vi "111 (SubVI).vi"(0 "scan angle":sgl=90.0, 5 "step angle":sgl=4.0, 7 "stop":bool) -> (2 "sensor":bool, 3 "x":dbl, 4 "Data Value Reference out":refnum<data-value>, 6 "left motor":bool, 8 "y":dbl, 10 "right motor":bool, 12 "Array":u32[][](array[colorbox]), 13 "velocity":dbl, 14 "sensor data":cluster{dbl[], dbl[]}(graph)={[-0.048166929668633715], [0.4724490056471417]})   [LabVIEW 2011]
uses:
  <vilib>/robotics/Navigation/shared/WorldMap/OccupancyGridWorldMap/NI_Robotics_OccupancyGridWorldMap.lvclass
  <vilib>/Platform/TimedLoop/XDataNode/timing_clust.ctl
  <vilib>/Platform/TimedLoop/XDataNode/nitl_modes.ctl
  <vilib>/Platform/TimedLoop/XDataNode/wakeup.ctl
  <vilib>/robotics/Starter Kit/2.0/9632 Host Interface/NI_Robotics_Starter Kit Host_9632_2.0.lvclass
  <vilib>/Utility/AngleManip/Degrees to Radians (Scalar SGL).vi
  <vilib>/robotics/Steering/Steering Frame/Apply Steering Frame Velocity to Motors.vi
  <vilib>/Utility/AngleManip/Degrees to Radians (Scalar DBL).vi
  <vilib>/robotics/Steering/Steering Frame/Get Steering Frame Velocity from Motors.vi
  <vilib>/Platform/TimedLoop/XDataNode/XDataNode.xnode
  <vilib>/Utility/AngleManip/NI_AngleManipulation.lvlib
  <vilib>/robotics/Utilities/Scan Angles/NI_Robotics_Scan Angles.lvlib
  <vilib>/robotics/Starter Kit/2.0/NI_Robotics_Starter Kit Host_2.0.lvlib
  <vilib>/Platform/TimedLoop/XDataNode/XDNodeRunTimeDep.lvlib
  <vilib>/robotics/Starter Kit/Host Interface/NI_Robotics_Starter Kit Host.lvclass
  <vilib>/robotics/Steering/Steering Frame/NI_Robotics_Steering Frame.lvclass
  <vilib>/ptbypt/NI_PtbyPt.lvlib
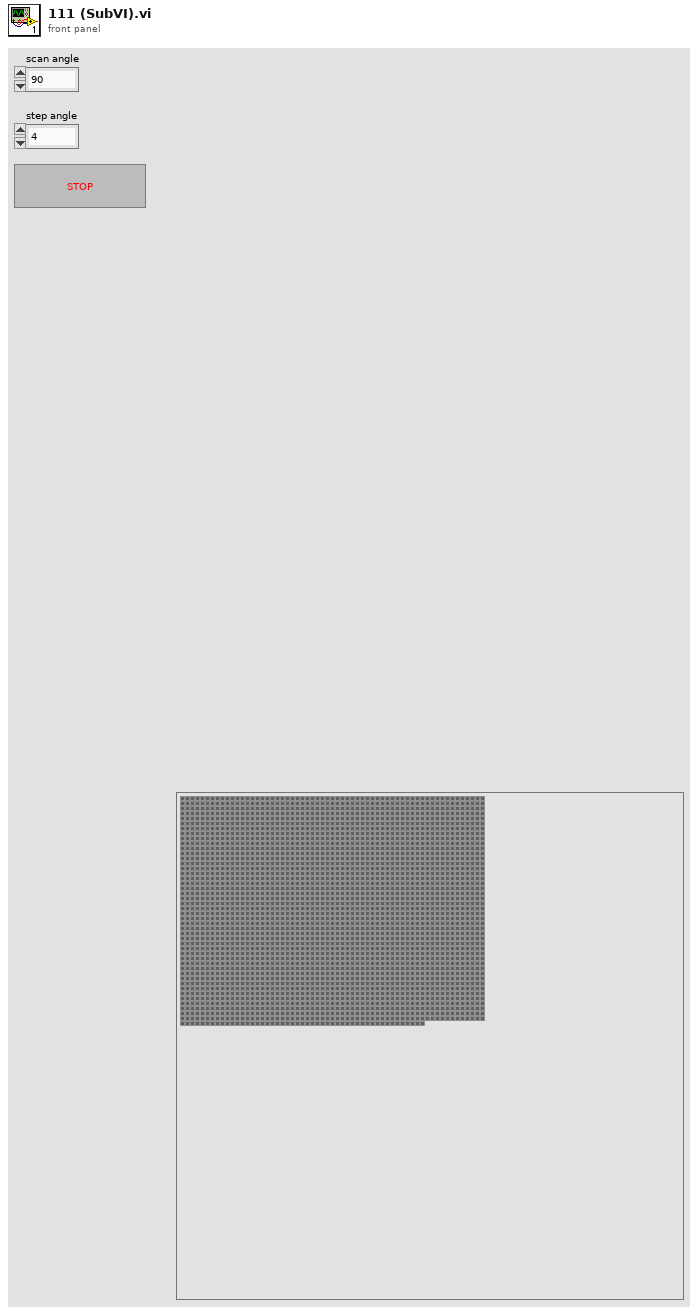
[diagram p1: front panel]
types:
  T1 = typedef "NI_Robotics_Scan Angles.lvlib/Scan Angle Data.ctl" = cluster{"angles":dbl[], "distances":dbl[], "current index":i32, "previous index":i32}
  T2 = typedef "XDNodeRunTimeDep.lvlib/timing_clust.ctl" = cluster{"Expected End [f-1]":u64, "Actual End [f-1]":u64, "Finished Late? [f-1]":bool, "Expected End [i-1]":u64, "Actual End [i-1]":u64, "Finished Late? [i-1]":bool, "Expected Start [i]":u64, "Actual Start [i]":u64, "Expected Start [f]":u64, "Actual Start [f]":u64, "Source Name":string, "Structure Name":string, "Period":i64, "Deadline":i64, "Offset":i64, "Start":i64, "Priority":i32, "Timeout":i32, "Mode":T3, "Wakeup Reason":T4, "Error":errorcluster, "Source Type":string, "Secondary Source Type":string, "Global End Time":u64, "Global Start Time":u64, "Frame Duration":u64, "Iteration Duration":u64, "Assigned CPU":i32, "I/O Scan Engine Mode":u32}
  T3 = typedef "XDNodeRunTimeDep.lvlib/nitl_modes.ctl" = enum32{"No Change", "Process missed periods, maintain original phase", "Discard missed periods, maintain original phase", "Process missed periods, ignore original phase", "Discard missed periods, ignore original phase"}
  T4 = typedef "XDNodeRunTimeDep.lvlib/wakeup.ctl" = enum32{"Normal", "Aborted", "Asynchronous wakeup", "Timing source error", "Timed loop error", "Timeout"}
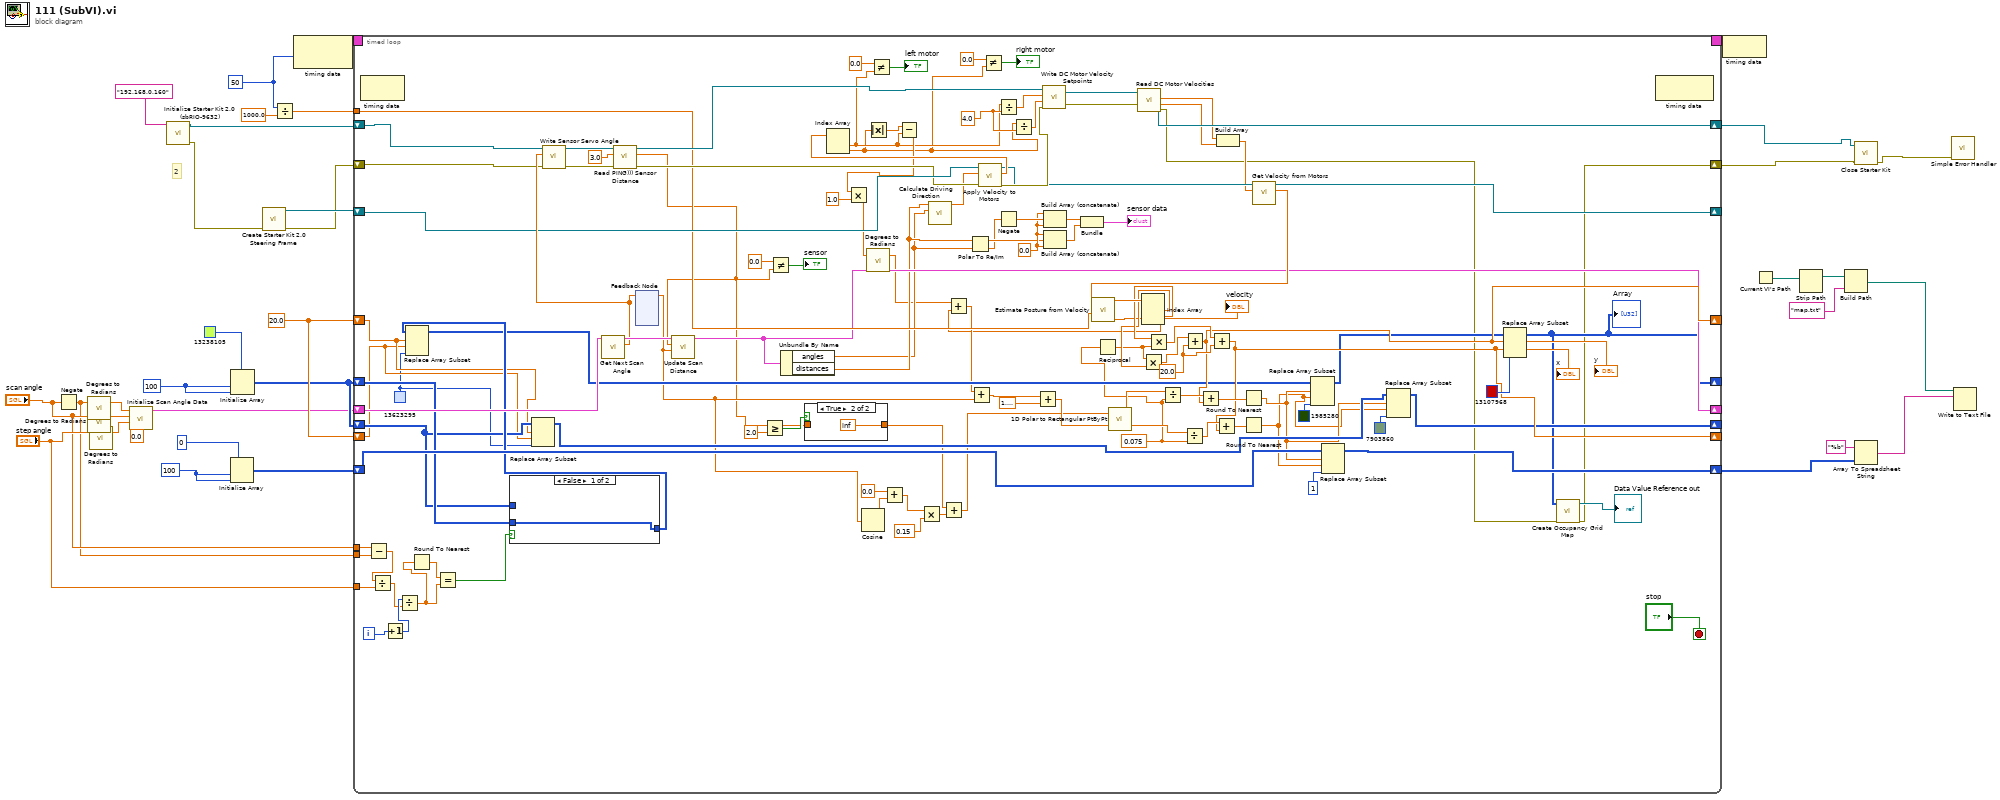
[diagram p0: block diagram]
diagram:
  w23 = 20.0
  w20 = i64 50 ("Period")
  w4 = 100 ("dimension size")
  w2 = 100 ("dimension size")
  # "2"
  n1 = Negate(x="scan angle") -> (-x=w31:sgl)
  n2 = call-poly <vilib>:"Degrees to Radians.vi"("angle (deg)"=w31) -> ("angle (rad)"=w6:sgl)  [unwired: 2 in]
  n3 = call-poly <vilib>:"Degrees to Radians.vi"("angle (deg)"="scan angle") -> ("angle (rad)"=w7:sgl)  [unwired: 2 in]
  n4 = call-poly <vilib>:"Degrees to Radians.vi"("angle (deg)"="step angle") -> ("angle (rad)"=w30:sgl)  [unwired: 2 in]
  n5 = call <vilib>:"Initialize Scan Angle Data.vi"("initial angle (0)"=0.0, "scan angle"=w30, "min angle"=w7, "max angle"=w6) -> ("scan angles"=w9:T1)  [unwired: 6 in, 1 out]
  n6 = call <vilib>:"Initialize Starter Kit 2.0 (sbRIO-9632).vi"("IP address (\"\")"="192.168.0.160" ("robot ID")) -> ("error out"=w25:errorcluster, "FPGA starter kit host 2.0 out"=w24:refnum<class "NI_Robotics_Starter Kit Host_9632_2.0.lvclass">)  [unwired: 9 in]
  n7 = Initialize Array(u32 0 ("element"), w4, w4) -> (w5:u32[][])
  n8 = Initialize Array(u32 13238105, w2, w2) -> (w22:u32[][])
  n9 = call <vilib>:"Create Starter Kit 2.0 Steering Frame.vi"("error in (no error)"=w25) -> ("error out"=w10:errorcluster, "starter kit differential steering frame"=w11:refnum<class "NI_Robotics_Differential Steering Frame.lvclass">)  [unwired: 9 in]
  n10 = Divide(x=w20, y=1000.0) -> (x/y=w21:dbl)
  n11 = node-c288(w20) -> (w35:T2)
  n12 = timed-loop {
    timing: w35 -> [_]
    timing-out: [_] -> w34
    shift-right: [w86] -> _
    shift-left: w9 -> [w143]
    shift-right: [w36] -> w28
    shift-left: w10 -> [w136]
    shift-right: [w150] -> w27
    shift-left: w24 -> [w135]
    shift-right: [w39] -> _
    shift-left: w22 -> [w107]
    shift-right: [w70] -> w17
    shift-left: w5 -> [w151]
    shift-right: [w128] -> _
    shift-left: w11 -> [w141]
    tunnel: w21 -> [w123]
    shift-right: [w112] -> _
    shift-left: w23 -> [w94]
    shift-right: [w111] -> _
    shift-left: w23 -> [w93]
    shift-right: [w103] -> _
    shift-left: w22 -> [w96]
    tunnel: w31 -> [w51]
    tunnel: "scan angle" -> [w50]
    tunnel: "step angle" -> [w49]
    i -> [w89]
    stop <- "stop" stop-if-true
    w83 = 0.0 ("element")
    w102 = 4.0 ("y")
    w92 = u32 13623295
    w120 = 20.0 ("y")
    w90 = 0.075 ("y")
    n13 = node-c288() -> ()  [unwired: 1 in, 1 out]
    n14 = Subtract(x=w50, y=w51) -> (x-y=w52:sgl)
    n15 = Divide(x=w52, y=w49) -> (x/y=w53:sgl)
    n16 = Increment(x=w89) -> (x+1=w88:i32)
    n17 = Divide(x=w88, y=w53) -> (x/y=w109:sgl)
    n18 = Round To Nearest(number=w109) -> (nearest integer value=w110:sgl)
    n19 = Equal?(x=w110, y=w109) -> (x = y?=w108:bool)
    n20 = case shown="False" w108 {
      tunnel: w107 -> [w154 _]
      tunnel: [w154 w155] -> w106
      tunnel: w96 -> [_ w155]
      frame False {
      }
      frame True {
      }
    }
    n21 = Replace Array Subset(array=w106, new element=w92, index (row)=w94, index (col)=w93) -> (w104:u32[][])
    n22 = Replace Array Subset(array=w96, new element=w92, index (row)=w94, index (col)=w93) -> (w95:u32[][])
    n23 = call <vilib>:"Get Next Scan Angle.vi"("scan angles in"=w143) -> ("new angle"=w144:dbl, "scan angles out"=w145:T1)  [unwired: 9 in]
    n24 = call <vilib>:"Write Sensor Servo Angle.vi"("error in (no error)"=w136, "ccw servo angle (rad)"=w144, "starter kit host in"=w135) -> ("error out"=w146:errorcluster, "starter kit host out"=w147:refnum<class "NI_Robotics_Starter Kit Host_9632_2.0.lvclass">)  [unwired: 7 in]
    n25 = call <vilib>:"Read PING))) Sensor Distance.vi"("error in (no error)"=w146, "default distance (NaN)"=3.0, "starter kit host in"=w147) -> ("error out"=w137:errorcluster, "distance (m)"=w40:dbl, "starter kit host out"=w138:refnum<class "NI_Robotics_Starter Kit Host_9632_2.0.lvclass">)  [unwired: 5 in, 1 out]
    n26 = feedback #1() -> (w54:dbl)  [unwired: 1 in]
    n27 = feedback-in #1(w144) -> ()
    n28 = call <vilib>:"Update Scan Distance.vi"("scan angle"=w54, "new scan distance"=w40, "scan angles in"=w145) -> ("scan angles out"=w86:T1)  [unwired: 8 in]
    n29 = Greater Or Equal?(x=w40, y=2.0) -> (x >= y?=w97:bool)
    n30 = Not Equal?(x=0.0, y=w40) -> (x != y?=→"sensor":bool)
    n31 = Unbundle By Name(w86) -> ("angles"=w75:dbl[], "distances"=w76:dbl[])
    n32 = case shown="True" w97 {
      tunnel: w40 -> [w152 _]
      tunnel: [w152 inf] -> w56
      frame False {
      }
      frame True {
      }
    }
    n33 = Cosine(x=w54) -> (cos(x)=w58:dbl)
    n34 = Add(x=0.0, y=w58) -> (x+y=w57:dbl)
    n35 = Multiply(x=w57, y=0.15) -> (x*y=w61:dbl)
    n36 = call "Calculate Driving Direction.vi"("obstacle angles (rad)"=w75, "obstacle distances (m)"=w76) -> ("steering frame velocity"=w74:dbl[])  [unwired: 8 in, 1 out]
    n37 = Add(x=w56, y=w61) -> (x+y=w55:dbl)
    n38 = Polar To Re/Im(2:w75, 3:w76) -> (0:w80:dbl[], 1:w81:dbl[])
    n39 = call-poly <vilib>:"Apply Velocity to Motors.vi"("error in (no error)"=w137, "steering frame velocity"=w74, "steering frame in"=w141) -> ("error out"=w139:errorcluster, "ccw motor velocity setpoints"=w140:dbl[], "steering frame out"=w127:refnum<class "NI_Robotics_Differential Steering Frame.lvclass">)  [unwired: 4 in, 2 out]
    n40 = Index Array(array=w140) -> (element #1=w46:dbl, element #2=w43:dbl)  [unwired: 2 in]
    n41 = Absolute Value(x=w43) -> (abs(x)=w69:dbl)
    n42 = Not Equal?(x=0.0, y=w46) -> (x != y?=→"left motor":bool)
    n43 = Subtract(x=w69, y=w46) -> (x-y=w65:dbl)
    n44 = Multiply(x=w65, y=1.0) -> (x*y=w63:dbl)
    n45 = call-poly <vilib>:"Degrees to Radians.vi"("angle (deg)"=w63) -> ("angle (rad)"=w66:dbl)  [unwired: 2 in]
    n46 = Not Equal?(x=0.0, y=w43) -> (x != y?=→"right motor":bool)
    n47 = Negate(x=w80) -> (-x=w85:dbl[])
    n48 = Divide(x=w46, y=w102) -> (x/y=w100:dbl)
    n49 = Divide(x=w43, y=w102) -> (x/y=w101:dbl)
    n50 = call <vilib>:"Write DC Motor Velocity Setpoints.vi"("error in (no error)"=w139, "right motor ccw velocity (rad/s)"=w101, "left motor ccw velocity (rad/s)"=w100, "starter kit host in"=w138) -> ("error out"=w148:errorcluster, "starter kit host out"=w149:refnum<class "NI_Robotics_Starter Kit Host_9632_2.0.lvclass">)  [unwired: 6 in]
    n51 = Build Array (concatenate)(w83, w85, w83) -> (w84:dbl[])
    n52 = Build Array (concatenate)(w83, w81, w83) -> (w82:dbl[])
    n53 = Bundle(w84, w82) -> (→"sensor data":cluster{dbl[], dbl[]})  [unwired: 1 in]
    n54 = Reciprocal(x=w90) -> (1/x=w91:dbl)
    n55 = call <vilib>:"Read DC Motor Velocities.vi"("error in (no error)"=w148, "starter kit host in"=w149) -> ("error out"=w37:errorcluster, "right motor ccw velocity (rad/s)"=w126:dbl, "left motor ccw velocity (rad/s)"=w125:dbl, "starter kit host out"=w150:refnum<class "NI_Robotics_Starter Kit Host_9632_2.0.lvclass">)  [unwired: 6 in]
    n56 = Build Array(w125, w126) -> (w124:dbl[])
    n57 = call-poly <vilib>:"Get Velocity from Motors.vi"("ccw motor velocity states"=w124, "steering frame in"=w127) -> ("estimated steering frame velocity"=w87:dbl[], "steering frame out"=w128:refnum<class "NI_Robotics_Differential Steering Frame.lvclass">)  [unwired: 7 in, 1 out]
    n58 = call "Estimate Posture from Velocity.vi"("dt (s)"=w123, "estimated steering frame velocity"=w87) -> ("y out"=→"velocity":dbl, "estimated steering frame posture"=w122:dbl[])  [unwired: 8 in]
    n59 = Index Array(array=w122) -> (element #1=w118:dbl, element #2=w119:dbl, element #3=w67:dbl)  [unwired: 3 in]
    n60 = Add(x=w66, y=w67) -> (x+y=w68:dbl)
    n61 = Add(x=w68, y=w54) -> (x+y=w77:dbl)
    n62 = Add(x=w77, y=1.5707963267948966) -> (x+y=w78:dbl)
    n63 = call <vilib>:"1D Polar to Rectangular PtByPt.vi"("phase"=w78, "magnitude"=w55) -> ("y"=w115:dbl, "x"=w114:dbl)
    n64 = Multiply(x=w91, y=w118) -> (x*y=w117:dbl)
    n65 = Multiply(x=w119, y=w91) -> (x*y=w116:dbl)
    n66 = Divide(x=w114, y=w90) -> (x/y=w134:dbl)
    n67 = Divide(x=w115, y=w90) -> (x/y=w130:dbl)
    n68 = Add(x=w117, y=w120) -> (x+y=w112:dbl)
    "y" <- w112
    n69 = Add(x=w134, y=w112) -> (x+y=w133:dbl)
    n70 = Add(x=w116, y=w120) -> (x+y=w111:dbl)
    "x" <- w111
    n71 = Add(x=w130, y=w111) -> (x+y=w129:dbl)
    n72 = Round To Nearest(number=w133) -> (nearest integer value=w73:dbl)
    n73 = Round To Nearest(number=w129) -> (nearest integer value=w72:dbl)
    n74 = Replace Array Subset(array=w104, new element=u32 1985280, index (row)=w73, index (col)=w72) -> (w71:u32[][])
    n75 = Replace Array Subset(array=w151, new element=u32 1 ("new element/subarray"), index (row)=w73, index (col)=w72) -> (w70:u32[][])
    n76 = Replace Array Subset(array=w95, new element=u32 7903860, index (row)=w73, index (col)=w72) -> (w103:u32[][])
    n77 = Replace Array Subset(array=w71, new element=u32 13107968, index (row)=w112, index (col)=w111) -> (w39:u32[][])
    "Array" <- w39
    n78 = call <vilib>:"Create Occupancy Grid Map.vi"("error in (no error)"=w37, "occupancy grid"=w39) -> ("error out"=w36:errorcluster, "map reference out"=→"Data Value Reference out":refnum<data-value>)  [unwired: 8 in]
    n79 = node-c288() -> ()  [unwired: 1 in, 1 out]
  }
  n80 = node-c288(w34) -> ()
  n81 = Current VI's Path() -> (path=w14:path)
  n82 = Strip Path(path=w14) -> (stripped path=w13:path)  [unwired: 1 out]
  n83 = Build Path(base path=w13, name or relative path="map.txt") -> (appended path=w15:path)
  n84 = call-dynamic "Close Starter Kit.vi"("error in (no error)"=w28, "starter kit host in"=w27) -> ("error out"=w29:errorcluster)  [unwired: 9 in]
  n85 = Array To Spreadsheet String(array=w17, 3:"%b" ("format string")) -> (spreadsheet string=w18:string)  [unwired: 1 in]
  n86 = call <vilib>:"Simple Error Handler.vi"("error in (no error)"=w29) -> ()  [unwired: 4 in, 5 out]
  n87 = Write to Text File(file (use dialog)=w15, text=w18) -> ()  [unwired: 2 in, 3 out]
